vi "MotherboardTest - TestStand - Get Termination Monitor Status.vi"(8 "error in (no error)":errorcluster, 11 "Status Monitor In":T1) -> (0 "error out":errorcluster, 2 "Terminating or Aborting":bool, 3 "Status Monitor Out":T1)   [LabVIEW 2013]
doc: "Monitors the execution that the VI is currently running in so the VI can stop if the user terminates or aborts the execution. Use this VI after you call the TestStand - Initialize Termination Monitor VI."
uses:
  MotherboardTest - TestStand - Status Monitor.ctl
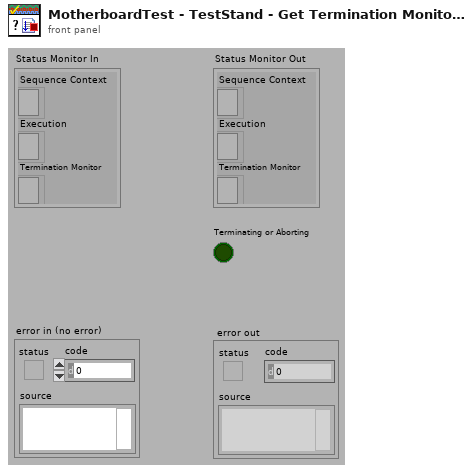
[diagram p1: front panel]
types:
  T1 = typedef "MotherboardTest - TestStand - Status Monitor.ctl" = cluster{"Sequence Context":refnum<k7>, "Execution":refnum<k7>, "Termination Monitor":refnum<k7>}
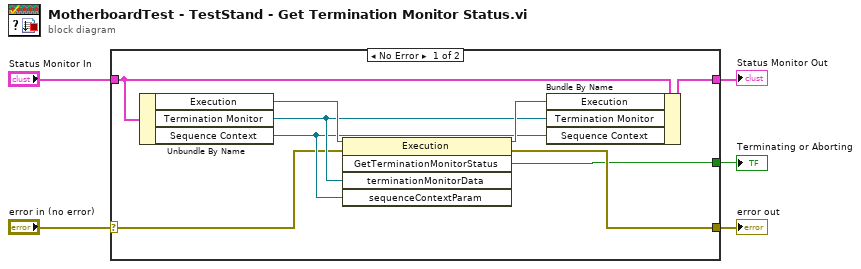
[diagram p0: block diagram]
diagram:
  n1 = case shown="No Error" "error in (no error)" {
    selector: "error in (no error)" -> [w6 w15]
    tunnel: [w14 w15] -> w5
    tunnel: [w13 w16] -> w4
    tunnel: "Status Monitor In" -> [w12 w16]
    tunnel: [w7 _] -> w2
    frame No Error {
      n2 = Unbundle By Name(w12) -> ("Execution"=w11:refnum<k7>, "Termination Monitor"=w9:refnum<k7>, "Sequence Context"=w8:refnum<k7>)
      n3 = invoke class="Execution" method="GetTerminationMonitorStatus"(reference=w11, error in=w6, "terminationMonitorData"=w9, "sequenceContextParam"=w8) -> (reference out=w10:refnum<k7>, error out=w14:errorcluster, "GetTerminationMonitorStatus"=w7:bool)  [unwired: 1 in, 2 out]
      n4 = Bundle By Name(cluster=w12, "Execution"=w10, "Termination Monitor"=w9, "Sequence Context"=w8) -> (w13:T1)
    }
    frame Error {
    }
  }
  "error out" <- w5
  "Status Monitor Out" <- w4
  "Terminating or Aborting" <- w2
